vi "force_control_daq.vi"() -> ()   [LabVIEW 2013]
uses:
  <resource>/objmgr/daqmx.rc
  <vilib>/DAQmx/create/channels.llb/DAQmx Create Channel (AI-Voltage-Basic).vi
  <vilib>/DAQmx/configure/timing.llb/DAQmx Timing (Sample Clock).vi
  <vilib>/Platform/TimedLoop/XDataNode/XDataNode.xnode
  <vilib>/Platform/TimedLoop/XDataNode/nitl_modes.ctl
  <vilib>/Platform/TimedLoop/XDataNode/XDNodeRunTimeDep.lvlib
  <vilib>/Platform/TimedLoop/XDataNode/wakeup.ctl
  <vilib>/Platform/TimedLoop/XDataNode/timing_clust.ctl
  <vilib>/Analysis/NI_AALBase.lvlib
  <vilib>/Analysis/baseanly.llb/Mean (DBL).vi
  <vilib>/DAQmx/read.llb/DAQmx Read (Analog 2D DBL NChan NSamp).vi
  <vilib>/Analysis/Matrix/NI_Matrix.lvlib
  <vilib>/Analysis/3filter.llb/Filter Passband Type.ctl
  force_control_globals.vi
  <vilib>/Analysis/Matrix/Numeric/Conversions/Matrix To Array - RM.vi
  <vilib>/ptbypt/NI_PtbyPt.lvlib
  <vilib>/Analysis/baseanly.llb/A x Vector.vi
panel:
  in  "FBG Rotation Angle (rad)":dbl=-0.0848
  in  "fl":i32=2
  in  "fh":i32=5
  in  "Fs":i32=1000
  in  "Accel Normal":dbl[](array[numeric])=[0.081638690183347, -0.359577292132026, 0.929537140327457]
  out "Saving":bool caption="Saving Data"
  in  "Log Data?":bool
  in  "Path":path=path "C:/data/FBG/fbg data log test.tdms"
  out "Load Cell Ref Output":dbl
  out "Load Cell Raw Output":dbl
  out "FBG Ref Output":dbl[](array[numeric])
  in  "Filter FBG":bool
  in  "Filter Load Cell":bool
  in  "Zero Load Cell":bool
  in  "Zero FBG":bool
  in  "Enable FBG":bool
  out "Load Cell Ref":dbl=1000.0
  out "FBG Refs":dbl[](array[numeric])
  in  "Enable Load Cell":bool
  out "FBG Output":dbl[](array[numeric])
  out "Accelerometer Output":dbl[][](array[numeric])
  out "Number of Sensors":u16[](array[numeric])
  in  "Stop Button":bool
  in  "Plane Normal":dbl[](array[numeric])=[-22489.0, -83132.0, -16505.0]
  in  "Use Plane Normal":bool
  in  "Accel Sample Rate":sgl=100.0 format="%0.2f"
  in  "Accel Sample Length":i32=100
  in  "Analog Data Test":dbl[](array[numeric])=[1.0, 2.0, 3.0, 4.0, 5.0, 6.0]
  out "Analog Data":dbl[](array[numeric])
  # "Load Cell Data"
  # "FBG Data"
  # "Accelerometer Data"
  # "Parameters"
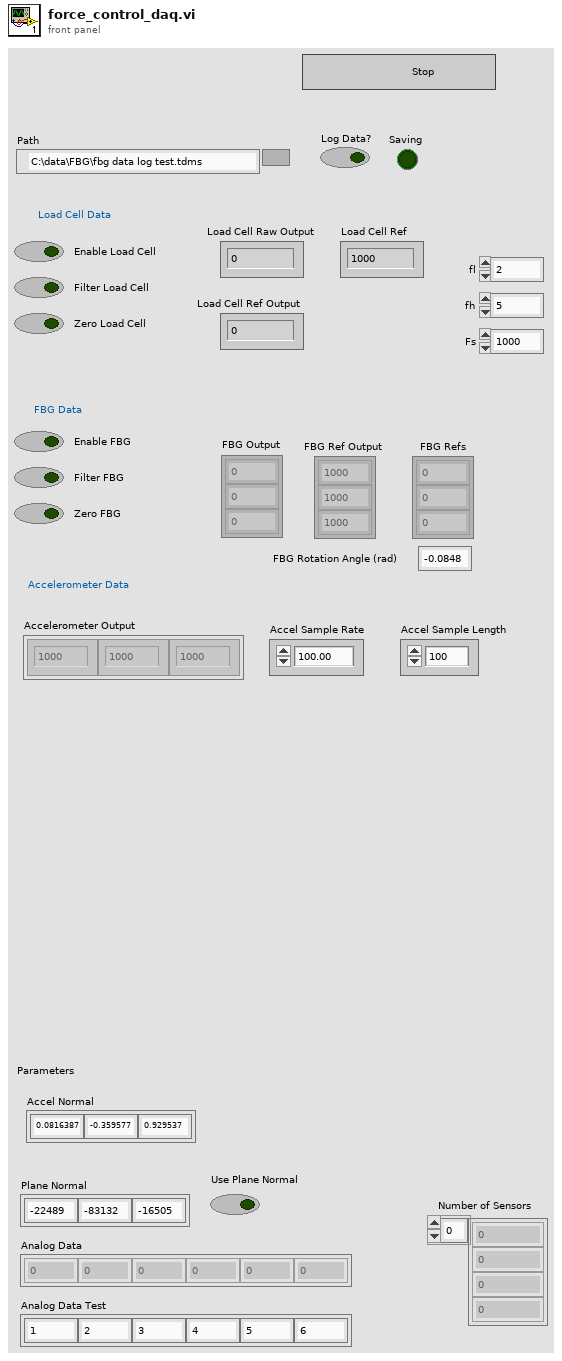
[diagram p1: front panel]
types:
  T1 = typedef "XDNodeRunTimeDep.lvlib/timing_clust.ctl" = cluster{"Expected End [f-1]":u64, "Actual End [f-1]":u64, "Finished Late? [f-1]":bool, "Expected End [i-1]":u64, "Actual End [i-1]":u64, "Finished Late? [i-1]":bool, "Expected Start [i]":u64, "Actual Start [i]":u64, "Expected Start [f]":u64, "Actual Start [f]":u64, "Source Name":string, "Structure Name":string, "Period":i64, "Deadline":i64, "Offset":i64, "Start":i64, "Priority":i32, "Timeout":i32, "Mode":T2, "Wakeup Reason":T3, "Error":errorcluster, "Source Type":string, "Secondary Source Type":string, "Global End Time":u64, "Global Start Time":u64, "Frame Duration":u64, "Iteration Duration":u64, "Assigned CPU":i32, "I/O Scan Engine Mode":u32}
  T2 = typedef "XDNodeRunTimeDep.lvlib/nitl_modes.ctl" = enum32{"No Change", "Process missed periods, maintain original phase", "Discard missed periods, maintain original phase", "Process missed periods, ignore original phase", "Discard missed periods, ignore original phase"}
  T3 = typedef "XDNodeRunTimeDep.lvlib/wakeup.ctl" = enum32{"Normal", "Aborted", "Asynchronous wakeup", "Timing source error", "Timed loop error", "Timeout"}
  T4 = typedef "NI_AALBase.lvlib/Filter Passband Type.ctl" = enum32{"Lowpass", "Highpass", "Bandpass", "Bandstop"}
  T5 = typedef "NI_Matrix.lvlib/RealMatrix.ctl" = dbl[][]
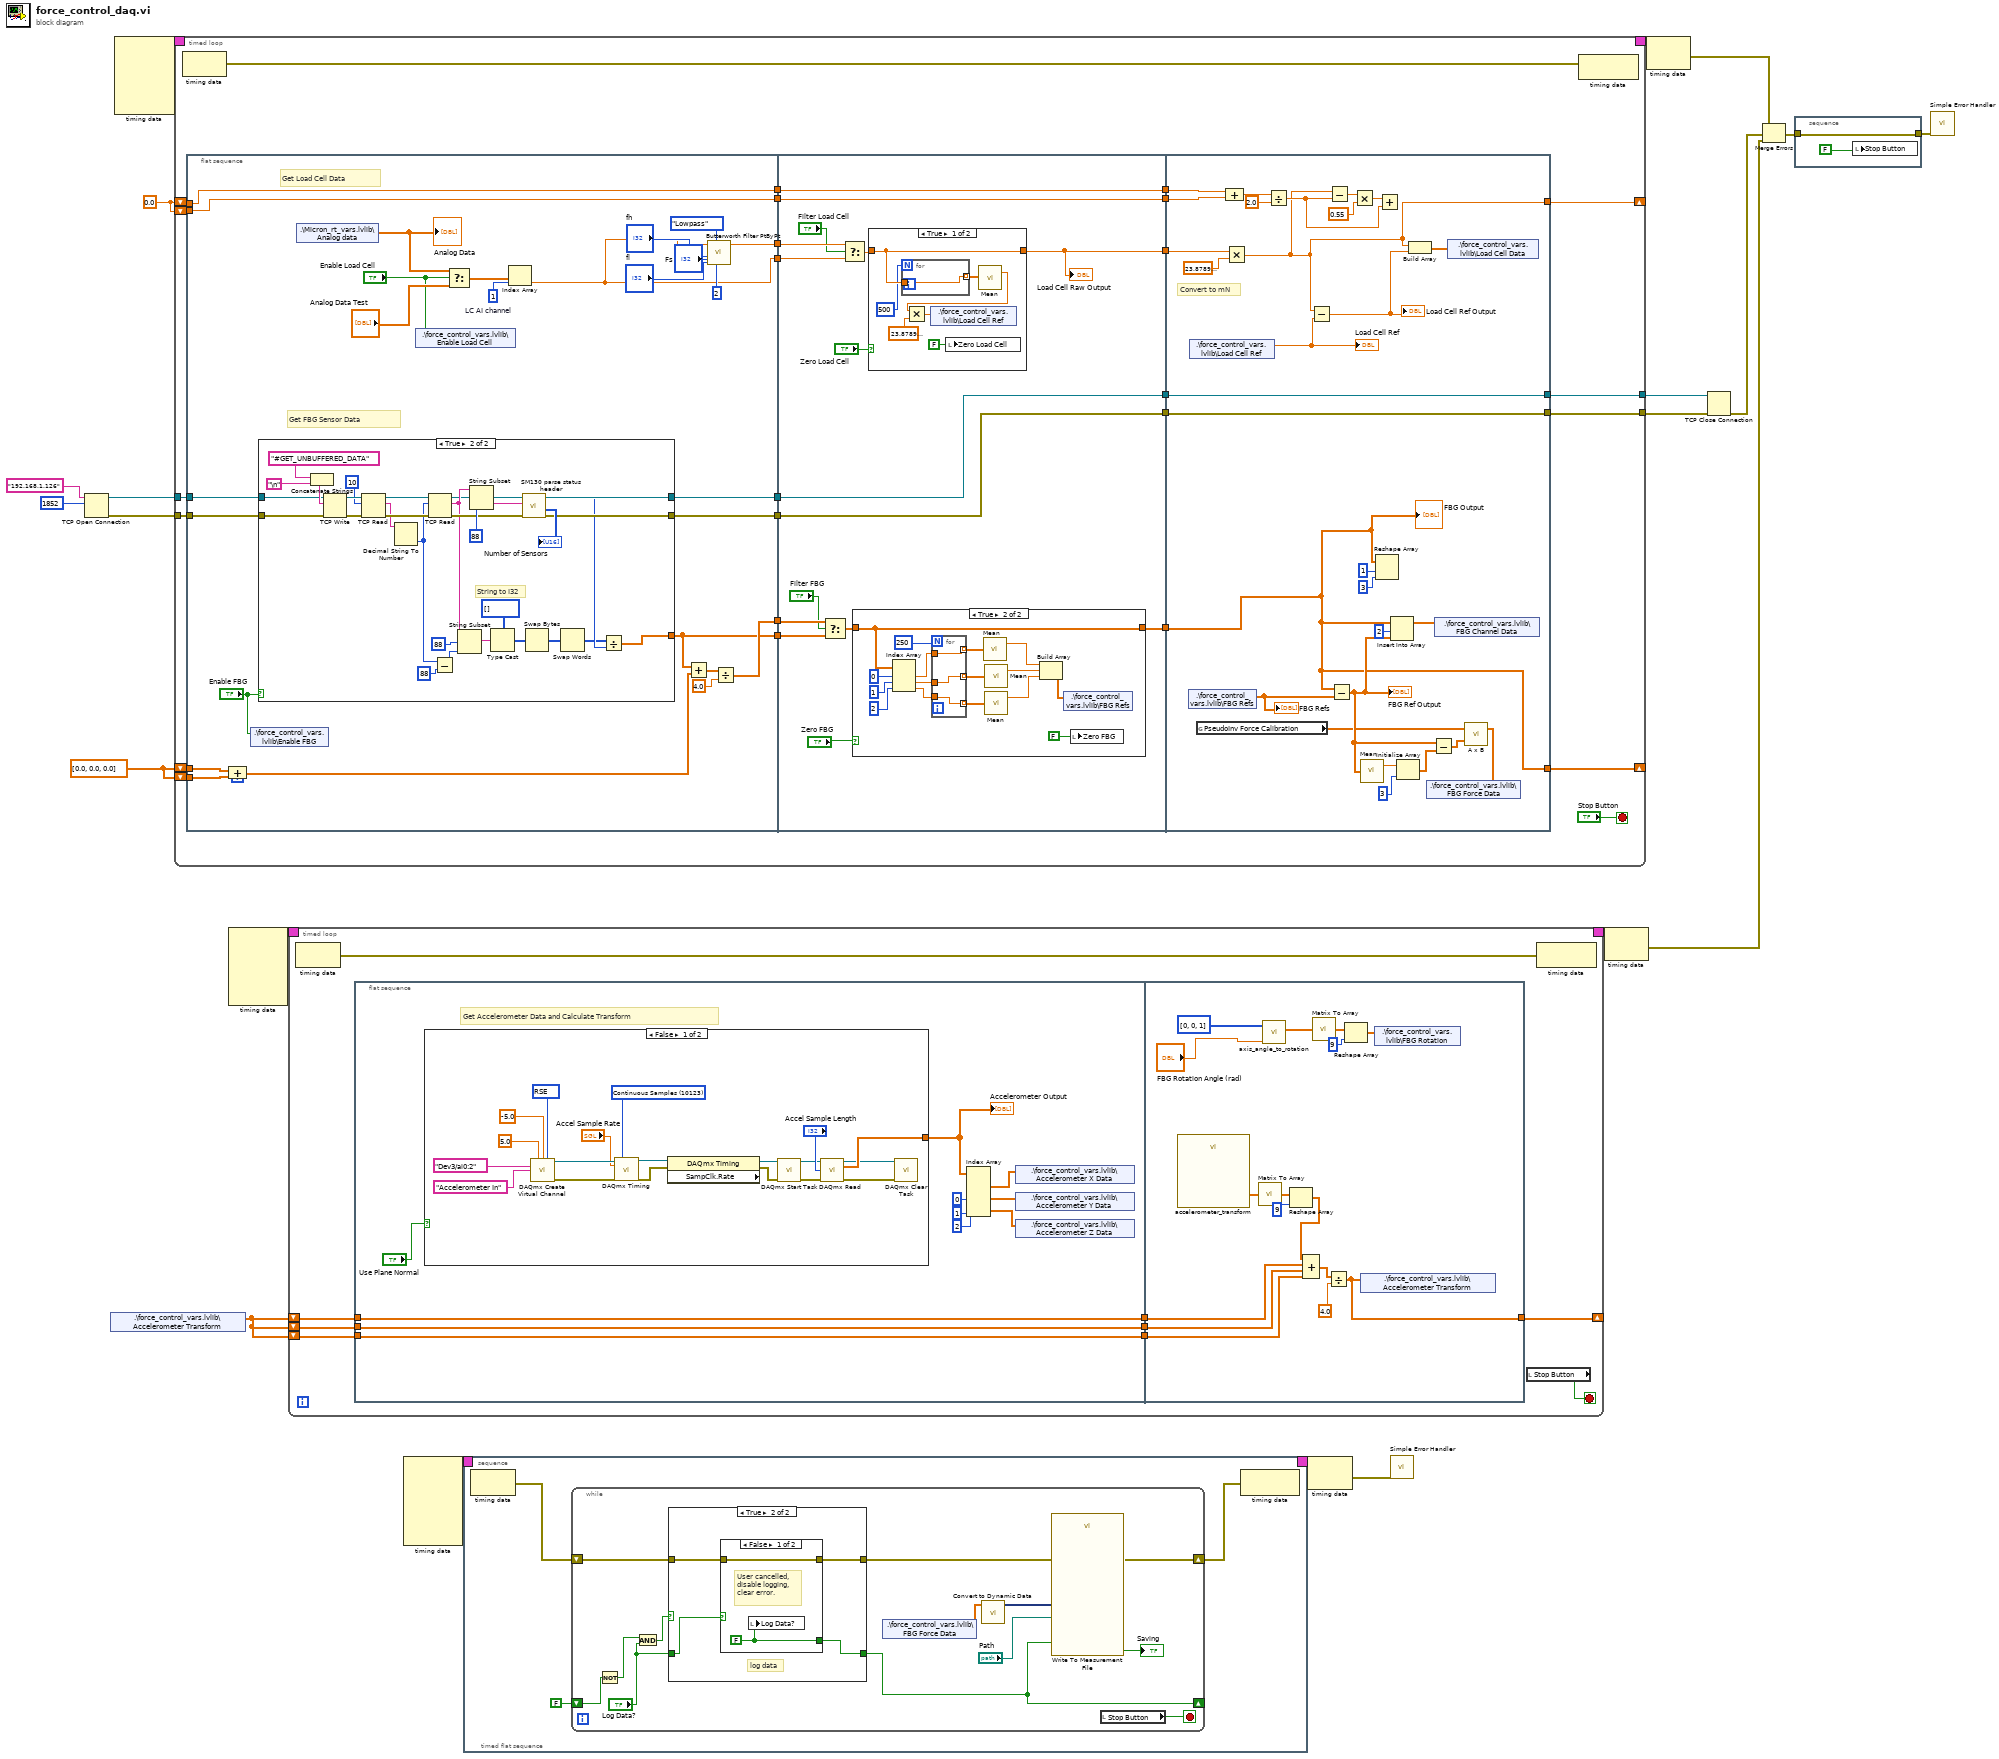
[diagram p0: block diagram]
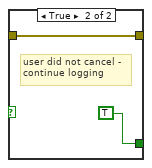
[diagram p3: hidden frame]
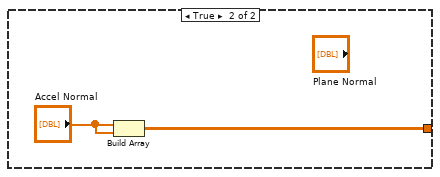
[diagram p4: hidden frame]
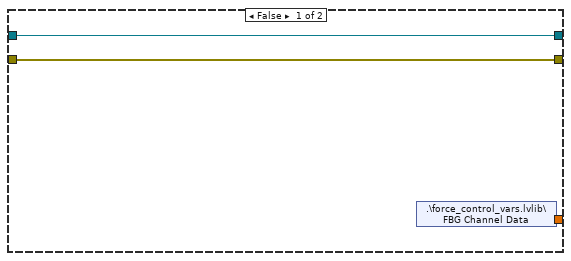
[diagram p5: hidden frame]
diagram:
  w1 = dbl[] [0.0, 0.0, 0.0]
  w2 = 0.0
  n1 = TCP Open Connection(address="192.168.1.126", remote port or service name=1852) -> (connection ID=w19:refnum<k5>, error out=w18:errorcluster)  [unwired: 3 in]
  n2 = shared-variable ".\\force_control_vars.lvlib\\Accelerometer Transform"() -> (w9:dbl[])  [unwired: 1 in, 1 out]
  n3 = node-c288() -> (w15:T1)  [unwired: 5 in]
  n4 = timed-loop {
    tunnel: w19 -> [w47]
    tunnel: w18 -> [w46]
    tunnel: [w45] -> w17
    tunnel: [w44] -> w16
    timing: w15 -> [_]
    timing-out: [_] -> w14
    shift-right: [w22] -> _
    shift-left: w2 -> [w38]
    shift-right: [w28] -> _
    shift-left: w1 -> [w42]
    shift-left: w1 -> [w43]
    shift-left: w2 -> [w39]
    stop <- "Stop Button" stop-if-true
    n5 = node-c288() -> (w40:errorcluster)  [unwired: 1 in]
    n6 = flat-sequence {
      tunnel: w47 -> [w73]
      tunnel: w46 -> [w72]
      tunnel: w43 -> [w63]
      tunnel: w42 -> [w62]
      tunnel: w39 -> [w55]
      tunnel: w38 -> [w56]
      tunnel: [w71] -> w37
      tunnel: [w70] -> w36
      tunnel: [w58] -> w35
      tunnel: [w57] -> w34
      tunnel: [w48] -> w33
      tunnel: [w52] -> w32
      tunnel: [w56] -> w25
      tunnel: [w55] -> w23
      tunnel: w37 -> [w121]
      tunnel: w36 -> [w120]
      tunnel: w35 -> [w113]
      tunnel: w34 -> [w112]
      tunnel: w33 -> [w116]
      tunnel: w32 -> [w117]
      tunnel: [w121] -> w31
      tunnel: [w120] -> w30
      tunnel: [w106] -> w29
      tunnel: [w111] -> w27
      tunnel: [w108] -> w26
      tunnel: w25 -> [w108]
      tunnel: [w107] -> w24
      tunnel: w23 -> [w107]
      tunnel: [w178] -> w44
      tunnel: [w179] -> w45
      tunnel: w31 -> [w179]
      tunnel: w30 -> [w178]
      tunnel: w29 -> [w153]
      tunnel: [w151] -> w28
      tunnel: w27 -> [w151]
      tunnel: [w152] -> w22
      tunnel: w26 -> [w156]
      tunnel: w24 -> [w155]
      frame #0 {
        w69 = 1  # LC AI channel
        # "Get FBG Sensor Data"
        # "Get Load Cell Data"
        n7 = Compound Arithmetic op=ADD(w62, w63) -> (w61:dbl[])
        n8 = shared-variable ".\\force_control_vars.lvlib\\Enable FBG"("Enable FBG") -> ()  [unwired: 1 in, 1 out]
        n9 = case shown="True" "Enable FBG" {
          tunnel: w73 -> [w76 w83]
          tunnel: w72 -> [w75 w82]
          tunnel: [w76 w81] -> w71
          tunnel: [w75 w80] -> w70
          tunnel: [w74 w77] -> w57
          frame False {
            n10 = shared-variable ".\\force_control_vars.lvlib\\FBG Channel Data"() -> (w74:dbl[])  [unwired: 1 in, 1 out]
          }
          frame True {
            # "String to I32"
            n11 = Concatenate Strings("#GET_UNBUFFERED_DATA", "\n") -> (w94:string)
            n12 = TCP Write(connection ID=w83, data in=w94, error in (no error)=w82) -> (connection ID out=w89:refnum<k5>, error out=w95:errorcluster)  [unwired: 1 in, 1 out]
            n13 = TCP Read(connection ID=w89, bytes to read=10, error in (no error)=w95) -> (connection ID out=w90:refnum<k5>, data out=w91:string, error out=w96:errorcluster)  [unwired: 2 in]
            n14 = Decimal String To Number(string=w91) -> (number=w85:i32)  [unwired: 2 in, 1 out]
            n15 = TCP Read(connection ID=w90, bytes to read=w85, error in (no error)=w96) -> (connection ID out=w81:refnum<k5>, data out=w84:string, error out=w87:errorcluster)  [unwired: 2 in]
            n16 = Subtract(x=w85, y=88) -> (x-y=w105:i32)
            n17 = String Subset(string=w84, offset (0)=88 ("length (rest)"), length (rest)=w105) -> (substring=w86:string)
            n18 = String Subset(string=w84, length (rest)=88 ("length (rest)")) -> (substring=w98:string)  [unwired: 1 in]
            n19 = Type Cast(type=i32[] [], x=w86) -> (*(type *) &x=w103:i32[])
            n20 = call "SM130 parse status header.vi"("error in (no error)"=w87, "Status Header In"=w98) -> ("error out"=w80:errorcluster, "Number of Sensors"=→"Number of Sensors":u16[], "Granularity"=w79:u32)  [unwired: 7 in]
            n21 = Swap Bytes(anything=w103) -> (byte swapped=w102:i32[])
            n22 = Swap Words(1:w102) -> (0:w78:i32[])
            n23 = Divide(x=w78, y=w79) -> (x/y=w77:dbl[])
          }
        }
        n24 = shared-variable ".\\Micron_rt_vars.lvlib\\Analog data"() -> (w66:sgl[])  [unwired: 2 out]
        "Analog Data" <- w66
        n25 = shared-variable ".\\force_control_vars.lvlib\\Enable Load Cell"("Enable Load Cell") -> ()  [unwired: 1 in, 1 out]
        n26 = Select(t=w66, s="Enable Load Cell", f="Analog Data Test") -> (s? t:f=w68:dbl[])
        n27 = Index Array(array=w68, index=w69) -> (element=w48:dbl)
        n28 = Add(x=w57, y=w61) -> (x+y=w60:dbl[])
        n29 = call <vilib>:"Butterworth Filter PtByPt.vi"("order"=2, "filter type"=Filter_Passband_Type."Lowpass", "low cutoff freq: fl"="fl", "high cutoff freq: fh"="fh", "sampling freq: fs"="Fs", "x"=w48) -> ("Filtered x"=w52:dbl)  [unwired: 3 in, 1 out]
        n30 = Divide(x=w60, y=4.0) -> (x/y=w58:dbl[])
      }
      frame #1 {
        n31 = Select(t=w113, s="Filter FBG", f=w112) -> (s? t:f=w115:dbl[])
        n32 = Select(t=w117, s="Filter Load Cell", f=w116) -> (s? t:f=w119:dbl)
        n33 = case shown="True" "Zero FBG" {
          tunnel: w115 -> [w122 w135]
          tunnel: [w122 w135] -> w111
          frame False {
          }
          frame True {
            n34 = Index Array(array=w135, index #1=0, index #2=1, index #3=2) -> (element #1=w130:dbl, element #2=w128:dbl, element #3=w126:dbl)
            n35 = for {
              N: 250 -> [_]
              tunnel: w130 -> [w141]
              tunnel: [w141] -> w129 mode=indexing
              tunnel: w128 -> [w140]
              tunnel: [w140] -> w127 mode=indexing
              tunnel: w126 -> [w139]
              tunnel: [w139] -> w125 mode=indexing
            }
            n36 = call-poly <vilib>:"Mean.vi"("X"=w129) -> ("mean"=w133:dbl)  [unwired: 1 out]
            n37 = call-poly <vilib>:"Mean.vi"("X"=w127) -> ("mean"=w134:dbl)  [unwired: 1 out]
            n38 = call-poly <vilib>:"Mean.vi"("X"=w125) -> ("mean"=w132:dbl)  [unwired: 1 out]
            n39 = Build Array(w133, w134, w132) -> (w124:dbl[])
            n40 = shared-variable ".\\force_control_vars.lvlib\\FBG Refs"(w124) -> ()  [unwired: 1 in, 1 out]
            n41 = local write "Zero FBG"(FALSE) -> ()
          }
        }
        n42 = case shown="True" "Zero Load Cell" {
          tunnel: w119 -> [w147 w150]
          tunnel: [w147 w150] -> w106
          frame True {
            n43 = for {
              N: 500 -> [_]
              tunnel: w147 -> [w149]
              tunnel: [w149] -> w145 mode=indexing
            }
            n44 = local write "Zero Load Cell"(FALSE) -> ()
            n45 = call-poly <vilib>:"Mean.vi"("X"=w145) -> ("mean"=w142:dbl)  [unwired: 1 out]
            n46 = Multiply(x=w142, y=sgl 23.879 ("Load Cell Conversion")) -> (x*y=w144:dbl)
            n47 = shared-variable ".\\force_control_vars.lvlib\\Load Cell Ref"(w144) -> ()  [unwired: 1 in, 1 out]
          }
          frame False {
          }
        }
        "Load Cell Raw Output" <- w106
      }
      frame #2 {
        # "Convert to mN"
        n48 = shared-variable ".\\force_control_vars.lvlib\\FBG Refs"() -> (w171:dbl[])  [unwired: 1 in, 1 out]
        "FBG Refs" <- w171
        n49 = shared-variable ".\\force_control_vars.lvlib\\Load Cell Ref"() -> (w175:dbl)  [unwired: 1 in, 1 out]
        "Load Cell Ref" <- w175
        n50 = global read "force_control_globals.vi" "PseudoInv Force Calibration"() -> (w168:dbl[][])
        n51 = Multiply(x=w153, y=sgl 23.879 ("Load Cell Conversion")) -> (x*y=w152:dbl)
        n52 = Compound Arithmetic op=ADD(w156, w155) -> (w161:dbl)
        n53 = Divide(x=w161, y=2.0) -> (x/y=w162:dbl)
        n54 = Subtract(x=w152, y=w175) -> (x-y=w176:dbl)
        "Load Cell Ref Output" <- w176
        n55 = Subtract(x=w152, y=w162) -> (x-y=w157:dbl)
        n56 = Subtract(x=w151, y=w171) -> (x-y=w172:dbl[])
        "FBG Ref Output" <- w172
        n57 = Multiply(x=w157, y=0.55 ("alpha")) -> (x*y=w159:dbl)
        n58 = call-poly <vilib>:"Mean.vi"("X"=w172) -> ("mean"=w166:dbl)  [unwired: 1 out]
        n59 = Reshape Array(w151, 1, 3) -> ()  [unwired: 1 out]
        n60 = Add(x=w159, y=w162) -> ()  [unwired: 1 out]
        n61 = Insert Into Array(array=w151, index=2, new element=w172) -> (w174:dbl[])
        n62 = Initialize Array(w166, 3) -> (w167:dbl[])
        n63 = Build Array(w152, w176) -> (w177:dbl[])
        n64 = Subtract(x=w172, y=w167) -> (x-y=w169:dbl[])
        n65 = shared-variable ".\\force_control_vars.lvlib\\FBG Channel Data"(w174) -> ()  [unwired: 1 in, 1 out]
        n66 = shared-variable ".\\force_control_vars.lvlib\\Load Cell Data"(w177) -> ()  [unwired: 1 in, 1 out]
        n67 = call-poly <vilib>:"A x B.vi"("Vector"=w169, "A"=w168) -> ("A x Vector"=w170:dbl[])  [unwired: 1 out]
        n68 = shared-variable ".\\force_control_vars.lvlib\\FBG Force Data"(w170) -> ()  [unwired: 1 in, 1 out]
        "FBG Output" <- w151
      }
    }
    n69 = node-c288(w40) -> ()  [unwired: 1 out]
  }
  n70 = node-c288() -> (w13:T1)  [unwired: 5 in]
  n71 = timed-loop {
    timing: w13 -> [_]
    timing-out: [_] -> w12
    shift-right: [w191] -> _
    shift-left: w9 -> [w190]
    shift-left: w9 -> [w189]
    shift-left: w9 -> [w188]
    stop <- w193 stop-if-true
    n72 = node-c288() -> (w192:errorcluster)  [unwired: 1 in]
    n73 = flat-sequence {
      tunnel: w190 -> [w196]
      tunnel: w189 -> [w195]
      tunnel: w188 -> [w194]
      tunnel: [w196] -> w187
      tunnel: [w195] -> w186
      tunnel: [w194] -> w185
      tunnel: [w235] -> w191
      tunnel: w187 -> [w234]
      tunnel: w186 -> [w233]
      tunnel: w185 -> [w232]
      frame #0 {
        # "Get Accelerometer Data and Calculate Transform"
        n74 = case shown="False" "Use Plane Normal" {
          tunnel: [w222 w224] -> w197
          frame False {
            w215 = 10123 items=["Finite Samples"=10178, "Continuous Samples"=10123, "Hardware Timed Single Point"=12522] ("Sample Mode")
            w211 = 10083 items=["default"=-1, "RSE"=10083, "NRSE"=10078, "Differential"=10106, "Pseudodifferential"=12529] ("Terminal Configuration")
            n75 = call-poly <vilib>:"DAQmx Create Virtual Channel.vi"("maximum value"=5.0 ("Max Voltage"), "minimum value"=-5.0 ("Min Voltage"), "input terminal configuration"=w211, "physical channels"=tag "Dev3/ai0:2" ("Physical Channel"), "name to assign"="Accelerometer In") -> ("task out"=w216:refnum<k21>, "error out"=w217:errorcluster)  [unwired: 9 in]
            n76 = call-poly <vilib>:"DAQmx Timing.vi"("task/channels in"=w216, "sample mode"=w215, "rate"="Accel Sample Rate", "error in"=w217) -> ("task out"=w220:refnum<k21>, "error out"=w221:errorcluster)  [unwired: 10 in]
            n77 = property class="DAQmx Timing" props=["SampClk.Rate"](reference=w220, error in=w221) -> (reference out=w218:refnum<k21>, error out=w219:errorcluster)  [unwired: 1 out]
            n78 = call <vilib>:"DAQmx Start Task.vi"("task/channels in"=w218, "error in"=w219) -> ("task out"=w208:refnum<k21>, "error out"=w207:errorcluster)  [unwired: 12 in]
            n79 = call-poly <vilib>:"DAQmx Read.vi"("task/channels in"=w208, "number of samples per channel"="Accel Sample Length", "error in"=w207) -> ("task out"=w206:refnum<k21>, "data"=w222:dbl[][], "error out"=w205:errorcluster)  [unwired: 10 in]
            n80 = call <vilib>:"DAQmx Clear Task.vi"("task in"=w206, "error in"=w205) -> ()  [unwired: 13 in, 1 out]
          }
          frame True {
            n81 = Build Array("Accel Normal", "Accel Normal") -> (w224:dbl[][])
          }
        }
        "Accelerometer Output" <- w197
        n82 = Index Array(array=w197, index (row) #1=0, index (row) #2=1, index (row) #3=2) -> (element #1=w198:dbl[], element #2=w199:dbl[], element #3=w200:dbl[])  [unwired: 3 in]
        n83 = shared-variable ".\\force_control_vars.lvlib\\Accelerometer X Data"(w198) -> ()  [unwired: 1 in, 1 out]
        n84 = shared-variable ".\\force_control_vars.lvlib\\Accelerometer Y Data"(w199) -> ()  [unwired: 1 in, 1 out]
        n85 = shared-variable ".\\force_control_vars.lvlib\\Accelerometer Z Data"(w200) -> ()  [unwired: 1 in, 1 out]
      }
      frame #1 {
        n86 = call "accelerometer_transform.vi"() -> ("ASAP to Surface rotation"=w236:T5)  [unwired: 11 in]
        n87 = call-poly <vilib>:"Matrix To Array.vi"("Real Matrix"=w236) -> ("Real 2D Array"=w237:dbl[][])
        n88 = call "axis_angle_to_rotation.vi"("Angle"="FBG Rotation Angle (rad)", "Axis"=i32[] [0, 0, 1]) -> ("Rotation"=w227:T5)  [unwired: 9 in]
        n89 = Reshape Array(w237, 9 ("dimension size")) -> (w241:dbl[])
        n90 = Compound Arithmetic op=ADD(w241, w234, w233, w232) -> (w239:dbl[])
        n91 = call-poly <vilib>:"Matrix To Array.vi"("Real Matrix"=w227) -> ("Real 2D Array"=w228:dbl[][])
        n92 = Divide(x=w239, y=4.0) -> (x/y=w235:dbl[])
        n93 = Reshape Array(w228, 9 ("dimension size")) -> (w230:dbl[])
        n94 = shared-variable ".\\force_control_vars.lvlib\\Accelerometer Transform"(w235) -> ()  [unwired: 1 in, 1 out]
        n95 = shared-variable ".\\force_control_vars.lvlib\\FBG Rotation"(w230) -> ()  [unwired: 1 in, 1 out]
      }
    }
    n96 = local read "Stop Button"() -> (w193:bool)
    n97 = node-c288(w192) -> ()  [unwired: 1 out]
  }
  n98 = node-c288() -> (w6:T1)  [unwired: 6 in]
  n99 = timed-sequence {
    timing: w6 -> [_]
    timing-out: [_] -> w5
    n100 = timed-flat-sequence {
      n101 = node-c288() -> (w248:errorcluster)  [unwired: 1 in]
      n102 = while {
        shift-right: [w257] -> _
        shift-left: FALSE ("Log?") -> [w260]
        shift-right: [w256] -> w247
        shift-left: w248 -> [w255]
        stop <- w250 stop-if-true
        n103 = Not(x=w260) -> (.not. x?=w261:bool)
        n104 = And(x=w261, y="Log Data?") -> (x .and. y?=w259:bool)
        n105 = case shown="True" w259 {
          tunnel: "Log Data?" -> [w264 w265]
          tunnel: [w264 w268] -> w257
          tunnel: [w263 w267] -> w254
          tunnel: w255 -> [w263 w266]
          frame False {
            # "do not log data"
          }
          frame True {
            # "log data"
            n106 = case shown="False" w265 {
              tunnel: [w270 TRUE ("Log?")] -> w268
              tunnel: w266 -> [w269 w272]
              tunnel: [w269 w272] -> w267
              frame False {
                w270 = FALSE ("Log?")
                # "User cancelled,\ndisable logging,\nclear error."
                n107 = local write "Log Data?"(w270) -> ()
              }
              frame True {
                # "user did not cancel - \ncontinue logging"
              }
            }
          }
        }
        n108 = shared-variable ".\\force_control_vars.lvlib\\FBG Force Data"() -> (w253:dbl[])  [unwired: 1 in, 1 out]
        n109 = call "Convert to Dynamic Data"("Array"=w253) -> ("Dynamic Data Type"=w252:dynamicdata)  [unwired: 3 in]
        n110 = call "Write To Measurement File"("Signals"=w252, "Enable"=w257, "error in (no error)"=w254, "Filename"="Path") -> ("Saving Data"=→"Saving":bool, "error out"=w256:errorcluster)  [unwired: 13 in, 1 out]
        n111 = local read "Stop Button"() -> (w250:bool)
      }
      n112 = node-c288(w247) -> ()  [unwired: 1 out]
    }
  }
  n113 = node-c288(w5) -> (w3:errorcluster)
  n114 = call <vilib>:"Simple Error Handler.vi"("error in (no error)"=w3) -> ()  [unwired: 1 in, 8 out]
  n115 = node-c288(w12) -> (w4:errorcluster)
  n116 = node-c288(w14) -> (w11:errorcluster)
  n117 = TCP Close Connection(connection ID=w17, error in (no error)=w16) -> (error out=w10:errorcluster)  [unwired: 1 in, 1 out]
  n118 = Merge Errors(w11, w10, w4) -> (w8:errorcluster)
  n119 = stacked-sequence {
    tunnel: [w278] -> w7
    tunnel: w8 -> [w278]
    frame #0 {
      n120 = local write "Stop Button"(FALSE) -> ()
    }
  }
  n121 = call <vilib>:"Simple Error Handler.vi"("error in (no error)"=w7) -> ()  [unwired: 1 in, 8 out]
